vi "TestGB.vi"(8 "errin":errorcluster, 10 "String":string) -> (0 "errout":errorcluster)   [LabVIEW 2020]
uses:
  <vilib>/regexp/Match Regular Expression.xnode
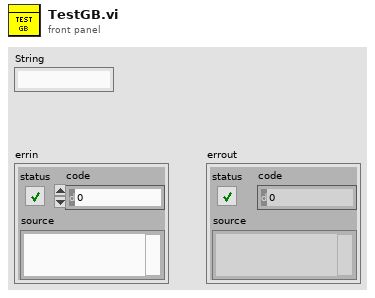
[diagram p1: front panel]
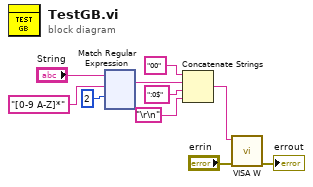
[diagram p0: block diagram]
diagram:
  n1 = xnode "Match Regular Expression"("chaîne en entrée"="String", "expression régulière"="[0-9 A-Z]*", "offset (0)"=2) -> ("toute l'expression"=w7:string)  [unwired: 3 in, 4 out]
  n2 = Concatenate Strings("00" ("chaîne"), w7, ":0$" ("chaîne"), "\r\n") -> (w3:string)
  n3 = call "VISA W.vi"("errin"="errin", "Chaîne"=w3) -> ("errout"=→"errout":errorcluster)  [unwired: 9 in]
